vi "ACP_LIMITS(LTE).vi"(0 "Session In":refnum<visa-resource-name>="TCPIP0::K-N90X0A-00005.local::hislip0::INSTR", 1 "Timeout":u32=3000, 11 "error in":errorcluster {"code" format="%.0x"}, 12 "BTS/MS":i32(ring) items=["MS"=1, "BTS"=0], 13 "REL/ABS":i32(ring) items=["ABS"=1, "REL"=0], 14 "INNER/OUTER":i32(ring) items=["OUTER"=1, "INNER"=0]) -> (4 "Session Out":refnum<visa-resource-name>="TCPIP0::K-N90X0A-00005.local::hislip0::INSTR", 6 "Limits":dbl[](array[numeric])=[-8.45, -8.45, -8.45, -8.45, -8.45, -8.45], 15 "error out":errorcluster {"code" format="%.0x"})   [LabVIEW 2018]
doc: "Launches the Instrument I/O Assistant, which you can use to communicate with message-based instruments and graphically parse the response. For example you can communicate with an instrument that uses a serial, Ethernet, or GPIB interface."
panel:
  # "READ ONLY VI  TO QUERY EXA MASK"
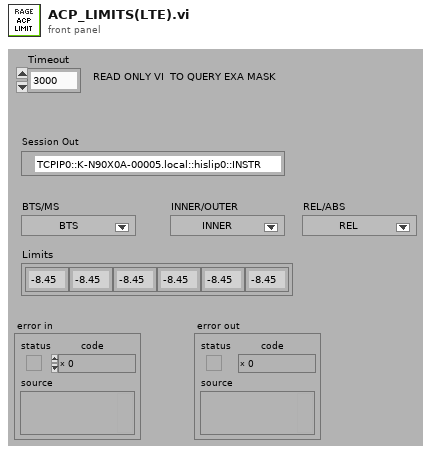
[diagram p1: front panel]
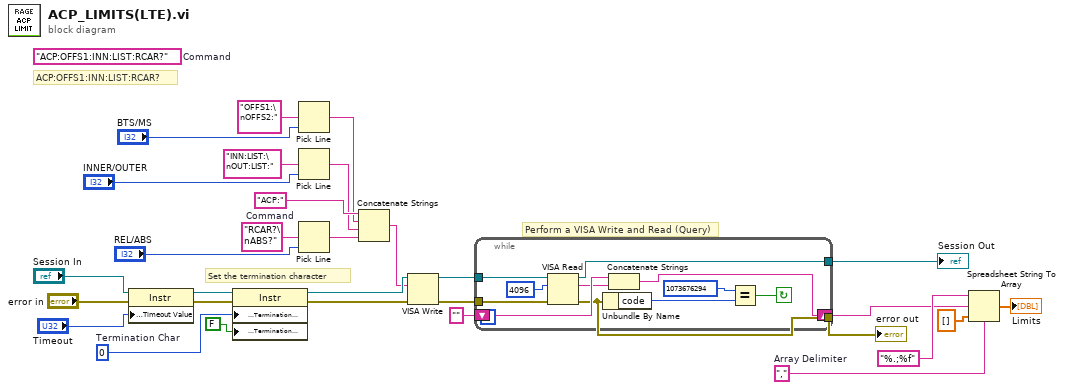
[diagram p0: block diagram]
diagram:
  (unwired) "ACP:OFFS1:INN:LIST:RCAR?"  # Command
  w16 = ","  # Array Delimiter
  w11 = "ACP:"  # Command
  w25 = u8 0  # Termination Char
  # "ACP:OFFS1:INN:LIST:RCAR?"
  # "Perform a VISA Write and Read (Query)"
  # "Set the termination character"
  n1 = property class="Instr"(reference="Session In", error in="error in", "General Settings:Timeout Value"="Timeout") -> (reference out=w24:refnum<visa-resource-name>, error out=w27:errorcluster)
  n2 = property class="Instr"(reference=w24, error in=w27, "Message Based Settings:Termination Character"=w25, "Message Based Settings:Termination Character Enable"=FALSE ("enable")) -> (reference out=w14:refnum<visa-resource-name>, error out=w26:errorcluster)
  n3 = Pick Line(multi-line string="OFFS1:\nOFFS2:", line index="BTS/MS") -> (output string=w8:string)  [unwired: 1 in]
  n4 = Pick Line(multi-line string="INN:LIST:\nOUT:LIST:", line index="INNER/OUTER") -> (output string=w4:string)  [unwired: 1 in]
  n5 = Pick Line(multi-line string="RCAR?\nABS?", line index="REL/ABS") -> (output string=w2:string)  [unwired: 1 in]
  n6 = Concatenate Strings(w11, w8, w4, w2) -> (w10:string)
  n7 = VISA Write(VISA resource name=w14, write buffer=w10, error in (no error)=w26) -> (VISA resource name out=w22:refnum<visa-resource-name>, error out=w21:errorcluster)  [unwired: 1 out]
  n8 = while {
    tunnel: w22 -> [w38]
    shift-right: [w32] -> w15
    shift-left: "" -> [w37]
    tunnel: w21 -> [w35]
    tunnel: [w34] -> w20
    tunnel: [w31] -> w13
    stop <- w33 continue-if-true
    n9 = VISA Read(VISA resource name=w38, byte count=u32 4096 ("byte count (0)"), error in (no error)=w35) -> (VISA resource name out=w31:refnum<visa-resource-name>, read buffer=w36:string, error out=w34:errorcluster)  [unwired: 1 out]
    n10 = Unbundle By Name(w34) -> ("code"=w40:i32)
    n11 = Concatenate Strings(w37, w36) -> (w32:string)
    n12 = Equal?(x=1073676294, y=w40) -> (x = y?=w33:bool)
  }
  "error out" <- w20
  "Session Out" <- w13
  n13 = Spreadsheet String To Array(delimiter (Tab)=w16, format string="%.;%f", spreadsheet string=w15, array type (2D Dbl)=dbl[] []) -> (array=→"Limits":dbl[])
